vi "Modify TIFF Image Description Tag.vi"() -> ()   [LabVIEW 2012]
doc: "SciScan 1.2 160622"
uses:
  Libtiff3/libtiff3.dll
panel:
  in  "ImageDescription":string
  out "error out":errorcluster
  in  "error in":errorcluster
  in  "path":path
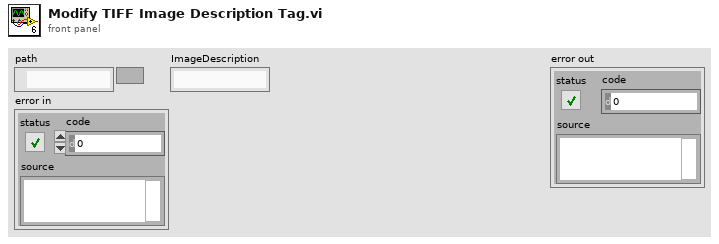
[diagram p1: front panel]
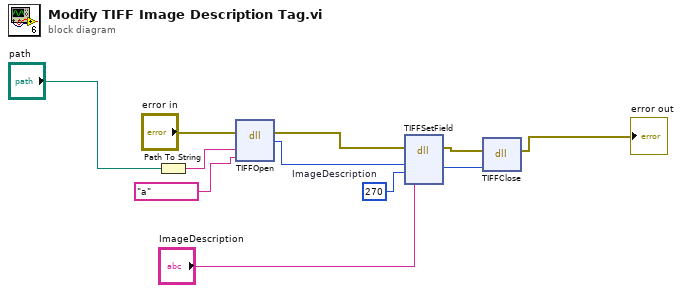
[diagram p0: block diagram]
diagram:
  w11 = 270  # ImageDescription
  n1 = Path To String(path="path") -> (string=w9:string)
  n2 = dll-call lib="D:/gitrepo/140812_ssdev_repo/Libtiff3/libtiff3.dll" fn="TIFFOpen"(error in="error in", "Filename"=w9, "Mode"="a") -> (error out=w5:errorcluster, w8:i32)  [unwired: 3 in, 2 out]
  n3 = dll-call lib="D:/gitrepo/140812_ssdev_repo/Libtiff3/libtiff3.dll" fn="TIFFSetField"(error in=w5, "Handle"=w8, "TIFF_tag"=w11, "Value"="ImageDescription") -> (error out=w4:errorcluster, "Handle"=w2:i32)  [unwired: 4 in, 2 out]
  n4 = dll-call lib="D:/gitrepo/140812_ssdev_repo/Libtiff3/libtiff3.dll" fn="TIFFClose"(error in=w4, "Handle"=w2) -> (error out=→"error out":errorcluster)  [unwired: 3 in, 2 out]
